vi "Result To Error.vi"(8 "error in (no error)":errorcluster, 11 "Result Code":i32) -> (0 "error out":errorcluster)   [LabVIEW 2020, in "G-Unicode.lvlib"]
doc: "Converts the result codes found in g_image.h to a custom LabVIEW error code. The custom error code range begins at 559513."
uses:
  G-Unicode.lvlib
  <vilib>/Utility/error.llb/Error Cluster From Error Code.vi
  <vilib>/ErrorRing/Error Ring.xnode
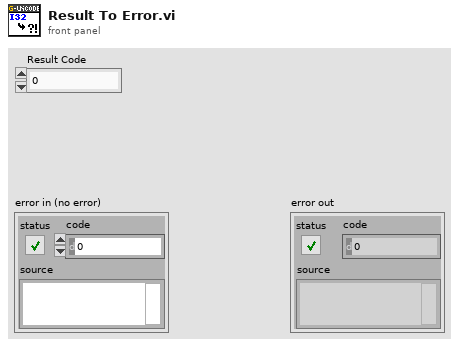
[diagram p1: front panel]
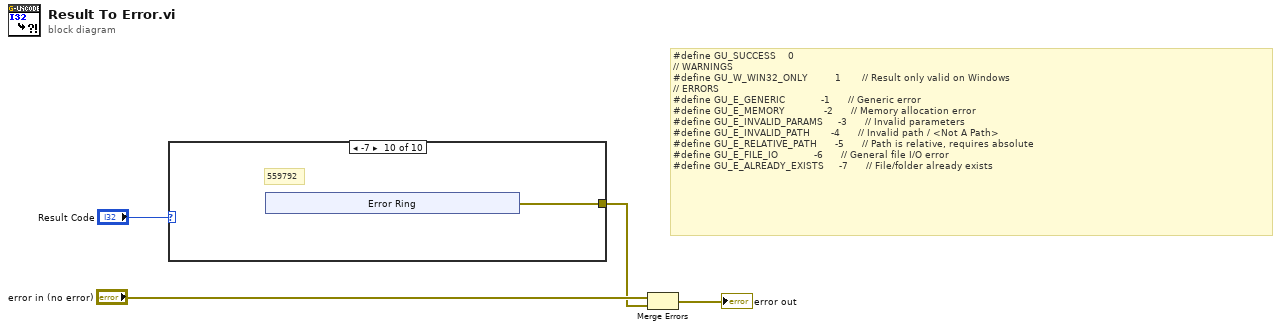
[diagram p0: block diagram]
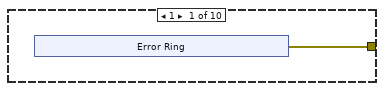
[diagram p2: hidden frame]
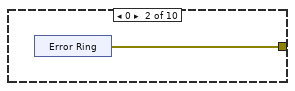
[diagram p3: hidden frame]
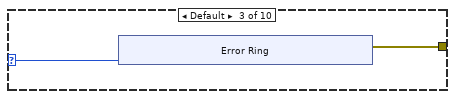
[diagram p4: hidden frame]
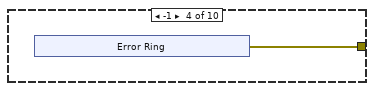
[diagram p5: hidden frame]
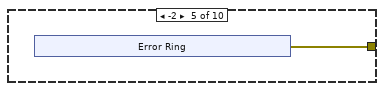
[diagram p6: hidden frame]
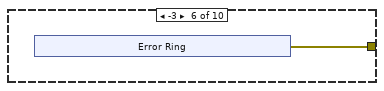
[diagram p7: hidden frame]
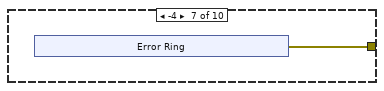
[diagram p8: hidden frame]
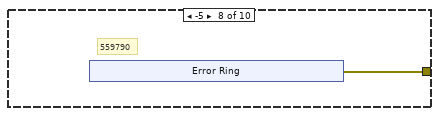
[diagram p9: hidden frame]
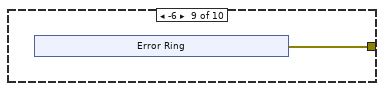
[diagram p10: hidden frame]
diagram:
  # "#define GU_SUCCESS\t\t\t\t0\n// WARNINGS\n#define GU_W_WIN32_ONLY         1       // Result only valid on Windows\n// ERRORS\n#define GU_E_GENERIC            -1      // Generic error\n#define GU_E_MEMORY             -2      // Memory allocation error\n#define GU_E_INVALID_PARAMS     -3      // Invalid parameters\n#define GU_E_INVALID_PATH       -4      // Invalid path / <Not A Path>\n#define GU_E_RELATIVE_PATH      -5      // Path is relative, requires absolute\n#define GU_E_FILE_IO            -6      // General file I/O error\n#define GU_E_ALREADY_EXISTS     -7      // File/folder already exists"
  n1 = case shown="-7" "Result Code" {
    selector: "Result Code" -> [_ _ w13 _ _ _ _ _ _ _]
    tunnel: [w5 w11 w14 w22 w28 w34 w40 w46 w51 w57] -> w1
    frame 1 {
      n2 = xnode "Error Ring"() -> ("error out"=w5:errorcluster)
    }
    frame 0 {
      n3 = xnode "Error Ring"() -> ("error out"=w11:errorcluster)
    }
    frame Default {
      n4 = xnode "Error Ring"("parameter 0"=w13) -> ("error out"=w14:errorcluster)
    }
    frame -1 {
      n5 = xnode "Error Ring"() -> ("error out"=w22:errorcluster)
    }
    frame -2 {
      n6 = xnode "Error Ring"() -> ("error out"=w28:errorcluster)
    }
    frame -3 {
      n7 = xnode "Error Ring"() -> ("error out"=w34:errorcluster)
    }
    frame -4 {
      n8 = xnode "Error Ring"() -> ("error out"=w40:errorcluster)
    }
    frame -5 {
      # "559790"
      n9 = xnode "Error Ring"() -> ("error out"=w46:errorcluster)
    }
    frame -6 {
      n10 = xnode "Error Ring"() -> ("error out"=w51:errorcluster)
    }
    frame -7 {
      # "559792"
      n11 = xnode "Error Ring"() -> ("error out"=w57:errorcluster)
    }
  }
  n12 = Merge Errors("error in (no error)", w1) -> (→"error out":errorcluster)
